vi "pomiar_czasu.vi"(6 "Reset":bool, 11 "czas do odmierzenia":dbl) -> (3 "gotowe":bool)   [LabVIEW 2025]
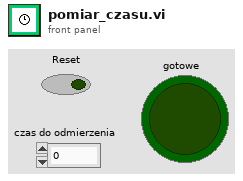
[diagram p1: front panel]
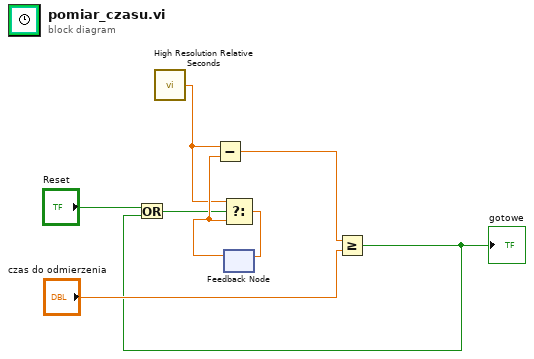
[diagram p0: block diagram]
diagram:
  n1 = call <vilib>:"High Resolution Relative Seconds.vi"() -> ("relative seconds"=w6:dbl)
  n2 = feedback #1() -> (w7:dbl)  [unwired: 1 in]
  n3 = Subtract(x=w6, y=w7) -> (x-y=w5:dbl)
  n4 = Greater Or Equal?(x=w5, y="czas do odmierzenia") -> (x >= y?=w1:bool)
  "gotowe" <- w1
  n5 = Or(x="Reset", y=w1) -> (x .or. y?=w2:bool)
  n6 = Select(t=w6, s=w2, f=w7) -> (s? t:f=w8:dbl)
  n7 = feedback-in #1(w8) -> ()
